vi "Controller X and Y to L and R Differential Drive.vi"(2 "Controller Y-Axis":dbl, 3 "Controller X-Axis":dbl) -> (0 "Right Side Motors":dbl, 1 "Left Side Motors":dbl)   [LabVIEW 2018]
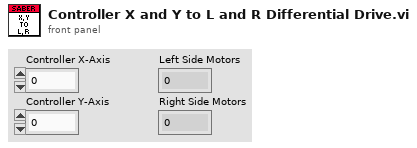
[diagram p1: front panel]
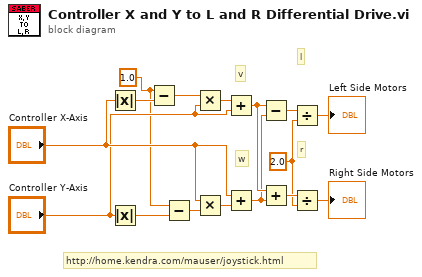
[diagram p0: block diagram]
diagram:
  w4 = 2.0 ("y")
  w1 = 1.0 ("s? t:f")
  # "http://home.kendra.com/mauser/joystick.html"
  # "r"
  # "l"
  # "w"
  # "v"
  n1 = Absolute Value(x="Controller X-Axis") -> (abs(x)=w16:dbl)
  n2 = Absolute Value(x="Controller Y-Axis") -> (abs(x)=w13:dbl)
  n3 = Subtract(x=w1, y=w16) -> (x-y=w15:dbl)
  n4 = Subtract(x=w1, y=w13) -> (x-y=w12:dbl)
  n5 = Multiply(x=w15, y="Controller Y-Axis") -> (x*y=w14:dbl)
  n6 = Multiply(x="Controller X-Axis", y=w12) -> (x*y=w11:dbl)
  n7 = Add(x=w14, y="Controller Y-Axis") -> (x+y=w9:dbl)
  n8 = Add(x="Controller X-Axis", y=w11) -> (x+y=w8:dbl)
  n9 = Subtract(x=w9, y=w8) -> (x-y=w10:dbl)
  n10 = Add(x=w9, y=w8) -> (x+y=w7:dbl)
  n11 = Divide(x=w10, y=w4) -> (x/y=→"Left Side Motors":dbl)
  n12 = Divide(x=w7, y=w4) -> (x/y=→"Right Side Motors":dbl)
